vi "incoming data.vi"(6 "timeout":i32=-1, 8 "error in":errorcluster, 9 "opcode":u8=1, 10 "data":string, 11 "Websocket console plugin in":refnum<class "Websocket console plugin.lvclass">) -> (0 "error out":errorcluster)   [LabVIEW 2013, in "Websocket console plugin.lvclass"]
uses:
  Websocket console plugin.lvclass
  Websocket console plugin.lvclass/Websocket console plugin.ctl
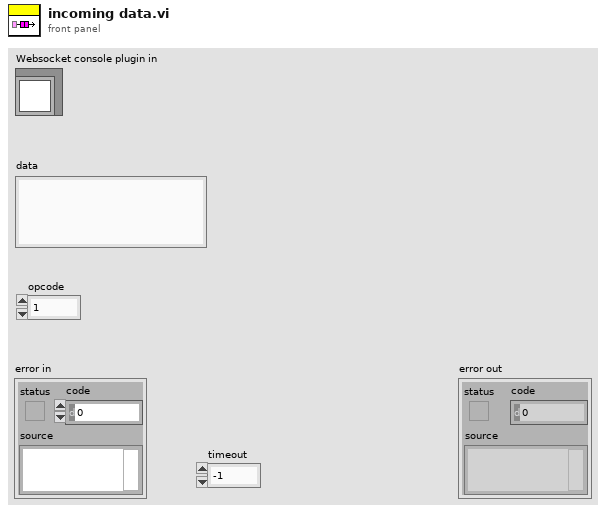
[diagram p1: front panel]
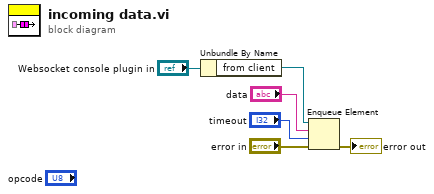
[diagram p0: block diagram]
diagram:
  n1 = Unbundle By Name("Websocket console plugin in") -> ("from client"=w2:refnum<queue>)
  n2 = Enqueue Element(queue=w2, element="data", timeout in ms (-1)="timeout", error in (no error)="error in") -> (error out=→"error out":errorcluster)  [unwired: 2 out]
